vi "FFT (multiple).vi"(8 "error in (no error)":errorcluster, 11 "XY-data":cluster{"X-array":dbl[], "Y-array":dbl[]}[](array[cluster]) {"Y-array" format="%.2p"; "X-array" format="%.2p"}) -> (0 "error out":errorcluster, 1 "phase []":cluster{"f0":dbl, "df":dbl, "phase":dbl[]}[](array[cluster]), 2 "magnitude []":cluster{"f0":dbl, "df":dbl, "magnitude":dbl[]}[](array[cluster]), 3 "XY-data out":cluster{"X-array":dbl[], "Y-array":dbl[]}[](array[cluster]) {"Y-array" format="%.2p"; "X-array" format="%.2p"})   [LabVIEW 2019, in "xy_utilities.lvlib"]
doc: "Computes the FFT spectrum of <B>XY-data</B>. This VI returns the FFT results as <B>magnitude</B> and <B>phase</B>. This VI is a wrapper for NI_MAPro.lvlib:FFT Spectrum (Mag-Phase).vi\n\nWire data to the data input to determine the polymorphic instance to use or manually select the instance."
uses:
  xy_utilities.lvlib
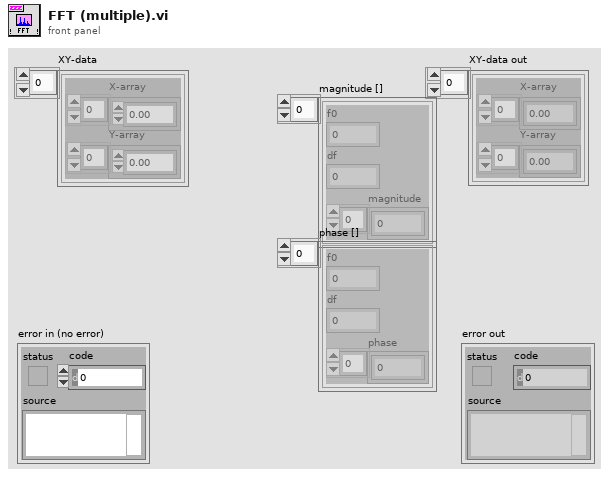
[diagram p1: front panel]
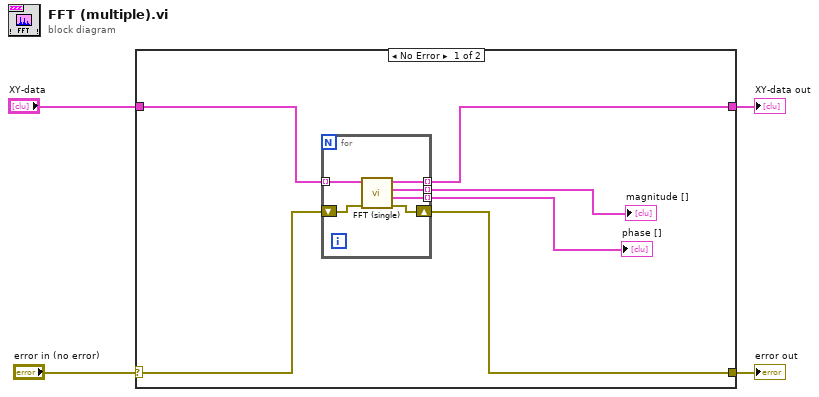
[diagram p0: block diagram]
diagram:
  n1 = case shown="No Error" "error in (no error)" {
    selector: "error in (no error)" -> [w6 w18]
    tunnel: [w5 w18] -> w3
    tunnel: "XY-data" -> [w10 w17]
    tunnel: [w9 w17] -> w1
    frame No Error {
      n2 = for {
        tunnel: w10 -> [w16] mode=indexing
        tunnel: [w15] -> w9 mode=indexing
        tunnel: [w14] -> w8 mode=indexing
        tunnel: [w11] -> w7 mode=indexing
        shift-right: [w13] -> w5
        shift-left: w6 -> [w12]
        n3 = call "FFT (single).vi"("error in (no error)"=w12, "XY-data"=w16) -> ("error out"=w13:errorcluster, "phase"=w11:cluster{"f0":dbl, "df":dbl, "phase":dbl[]}, "magnitude"=w14:cluster{"f0":dbl, "df":dbl, "magnitude":dbl[]}, "XY-data out"=w15:cluster{"X-array":dbl[], "Y-array":dbl[]})  [unwired: 6 in]
      }
      "magnitude []" <- w8
      "phase []" <- w7
    }
    frame Error {
    }
  }
  "error out" <- w3
  "XY-data out" <- w1
